vi "ManageSettings.vi"(8 "error in (no error)":errorcluster, 10 "Mode":enum16{"GET", "SET"}(ring), 11 "File Path":path) -> (0 "error out":errorcluster, 3 "File Path Out":path)   [LabVIEW 2019, in "ByteLVDevEnv.lvlib"]
uses:
  ByteLVDevEnv.lvlib
  <vilib>/Utility/sysdir.llb/System Directory Type.ctl
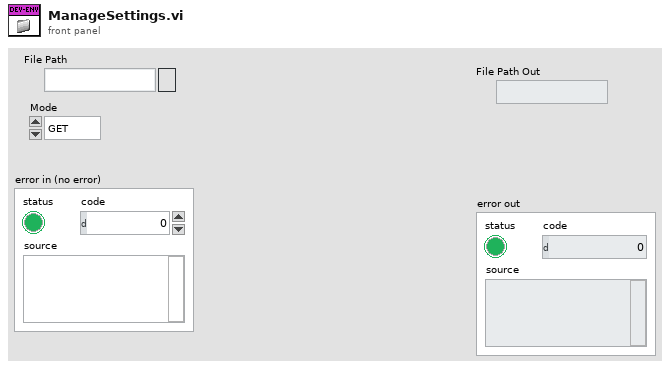
[diagram p1: front panel]
types:
  T1 = enum16{"open", "replace", "create", "open or create", "replace or create", "replace or create with confirmation"}
  T2 = typedef "System Directory Type.ctl" = i32
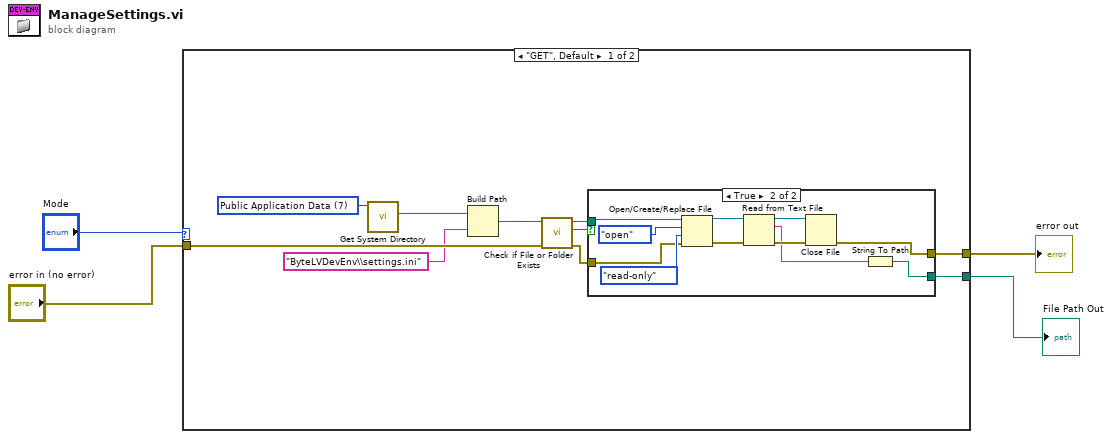
[diagram p0: block diagram]
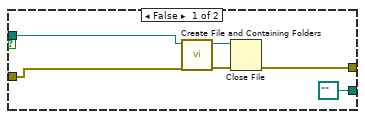
[diagram p2: hidden frame]
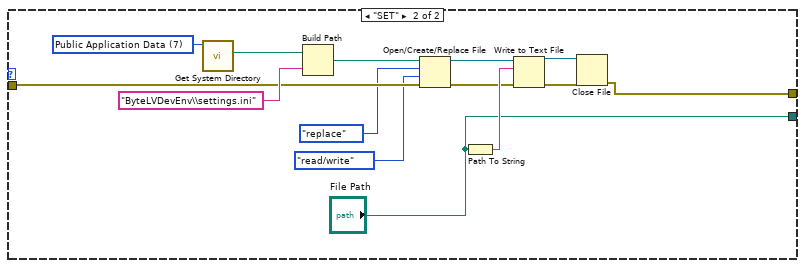
[diagram p3: hidden frame]
diagram:
  n1 = case shown="\"GET\", Default" "Mode" {
    tunnel: [w14 w33] -> w4
    tunnel: "error in (no error)" -> [w13 w41]
    tunnel: [w12 "File Path"] -> w2
    frame "GET", Default {
      w5 = T2 7 items=["User Home"=0, "User Desktop"=1, "User Documents"=2, "User Application Data"=3, "User Preferences"=4, "User Temporary"=5, "Public Documents"=6, "Public Application Data"=7, "Public Preferences"=8, "Public Cache"=13, "System Core Libraries"=9, "System Installed Libraries"=10, "Application Files"=11, "Boot Volume Root"=12] ("system directory type")
      n2 = call <vilib>:"Get System Directory.vi"("system directory type"=w5) -> ("system directory"=w6:path)  [unwired: 10 in]
      n3 = Build Path(base path=w6, name or relative path="ByteLVDevEnv\\settings.ini") -> (appended path=w7:path)
      n4 = call <vilib>:"Check if File or Folder Exists.vi"("error in (no error)"=w13, "path"=w7) -> ("error out"=w11:errorcluster, "file or folder exists?"=w8:bool, "dup path"=w9:path)  [unwired: 7 in]
      n5 = case shown="True" w8 {
        tunnel: w9 -> [w19 w31]
        tunnel: w11 -> [w20 w28]
        tunnel: [path "" w22] -> w12
        tunnel: [w15 w21] -> w14
        frame False {
          n6 = call <vilib>:"Create File and Containing Folders.vi"("error in (no error)"=w20, "file path"=w19) -> ("error out"=w17:errorcluster, "refnum out"=w16:refnum<file>)  [unwired: 8 in]
          n7 = Close File(refnum=w16, error in=w17) -> (error out=w15:errorcluster)  [unwired: 1 out]
        }
        frame True {
          n8 = Open/Create/Replace File(file path (use dialog)=w31, error in=w28, operation (0:open)=T1."open", access (0:read/write)=enum16{"read/write", "read-only", "write-only"}."read-only") -> (refnum out=w27:refnum<file>, error out=w26:errorcluster)  [unwired: 2 in, 1 out]
          n9 = Read from Text File(file (use dialog)=w27, error in=w26) -> (refnum out=w25:refnum<file>, text=w23:string, error out=w24:errorcluster)  [unwired: 2 in, 1 out]
          n10 = Close File(refnum=w25, error in=w24) -> (error out=w21:errorcluster)  [unwired: 1 out]
          n11 = String To Path(string=w23) -> (path=w22:path)
        }
      }
    }
    frame "SET" {
      w43 = T2 7 items=["User Home"=0, "User Desktop"=1, "User Documents"=2, "User Application Data"=3, "User Preferences"=4, "User Temporary"=5, "Public Documents"=6, "Public Application Data"=7, "Public Preferences"=8, "Public Cache"=13, "System Core Libraries"=9, "System Installed Libraries"=10, "Application Files"=11, "Boot Volume Root"=12] ("system directory type")
      n12 = call <vilib>:"Get System Directory.vi"("system directory type"=w43) -> ("system directory"=w44:path)  [unwired: 10 in]
      n13 = Build Path(base path=w44, name or relative path="ByteLVDevEnv\\settings.ini") -> (appended path=w42:path)
      n14 = Open/Create/Replace File(file path (use dialog)=w42, error in=w41, operation (0:open)=T1."replace", access (0:read/write)=enum16{"read/write", "read-only", "write-only"}."read/write") -> (refnum out=w38:refnum<file>, error out=w36:errorcluster)  [unwired: 2 in, 1 out]
      n15 = Path To String(path="File Path") -> (string=w37:string)
      n16 = Write to Text File(file (use dialog)=w38, text=w37, error in=w36) -> (refnum out=w35:refnum<file>, error out=w34:errorcluster)  [unwired: 1 in, 1 out]
      n17 = Close File(refnum=w35, error in=w34) -> (error out=w33:errorcluster)  [unwired: 1 out]
    }
  }
  "error out" <- w4
  "File Path Out" <- w2
